vi "Main.vi"() -> ()   [LabVIEW 2015]
uses:
  TypeDefs/Queue Data.ctl
  SubVIs/App Data.vi
  SubVIs/App Strings.vi
  FGV/Timer Actions.ctl
  Global 1.vi
panel:
  out "Status 3":string
  out "Status 2":string
  in  "Period [s]":dbl
  in  "Device name":tag="myDAQ1"
  out "Time Elapsed":dbl format="%<%M:%S>t"
  out "Status":string
  in  "Time [ms]":dbl
  in  "Frequency":dbl
  in  "Stop Button":bool
  in  "Acquire Button":bool
  out "Waveform Graph":dbl[](graph)
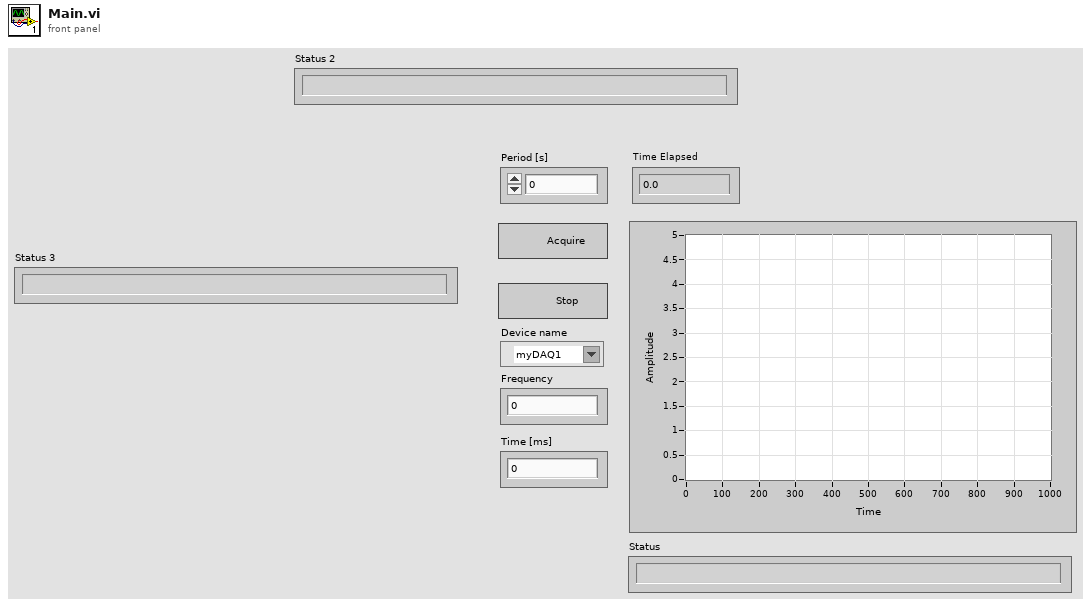
[diagram p1: front panel]
types:
  T1 = typedef "Timer Actions.ctl" = enum16{"Reset", "Get"}
  T2 = typedef "Queue Data.ctl" = cluster{"Action":string}
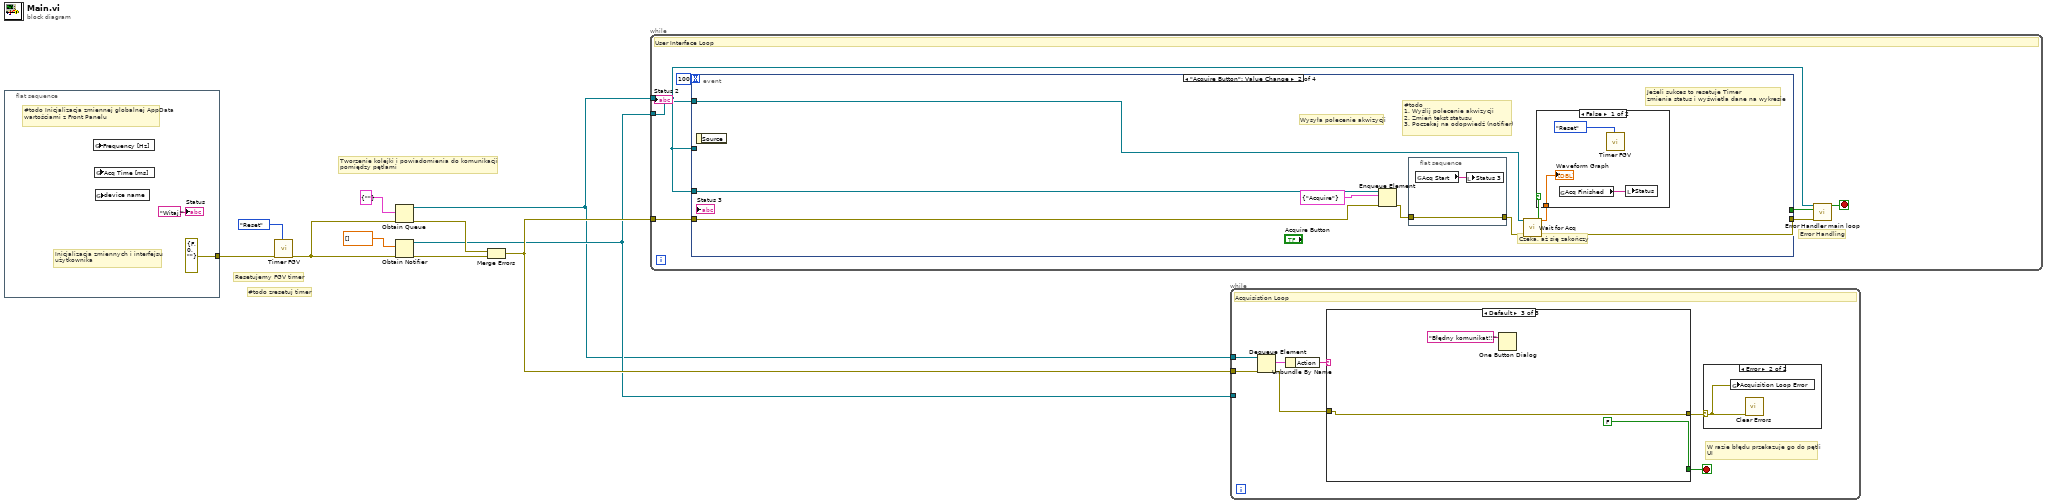
[diagram p0: block diagram]
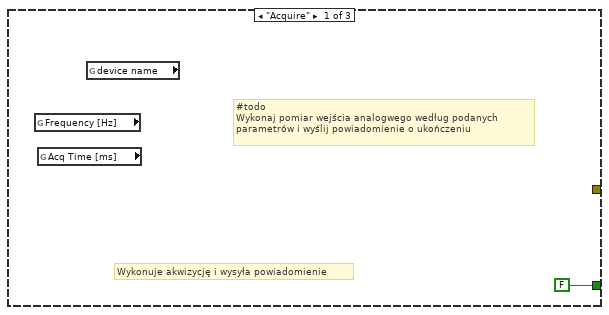
[diagram p3: hidden frame]
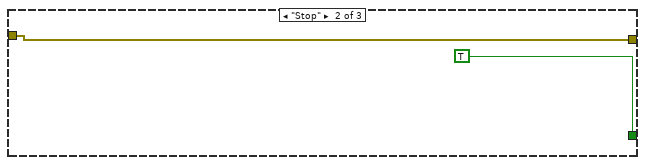
[diagram p4: hidden frame]
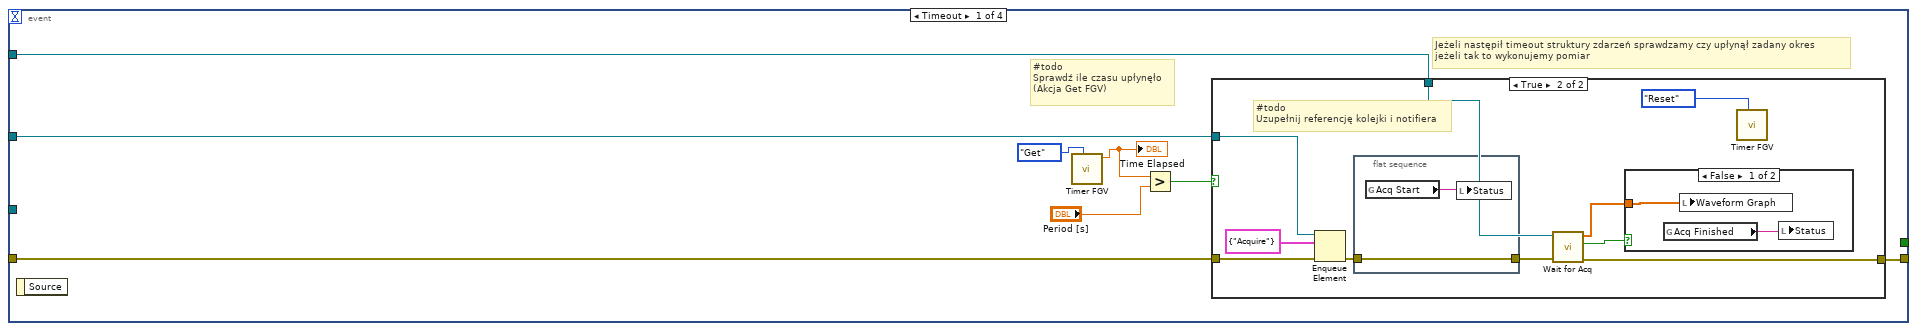
[diagram p5: hidden frame]
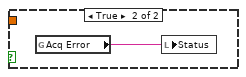
[diagram p7: hidden frame]
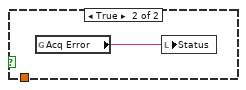
[diagram p8: hidden frame]
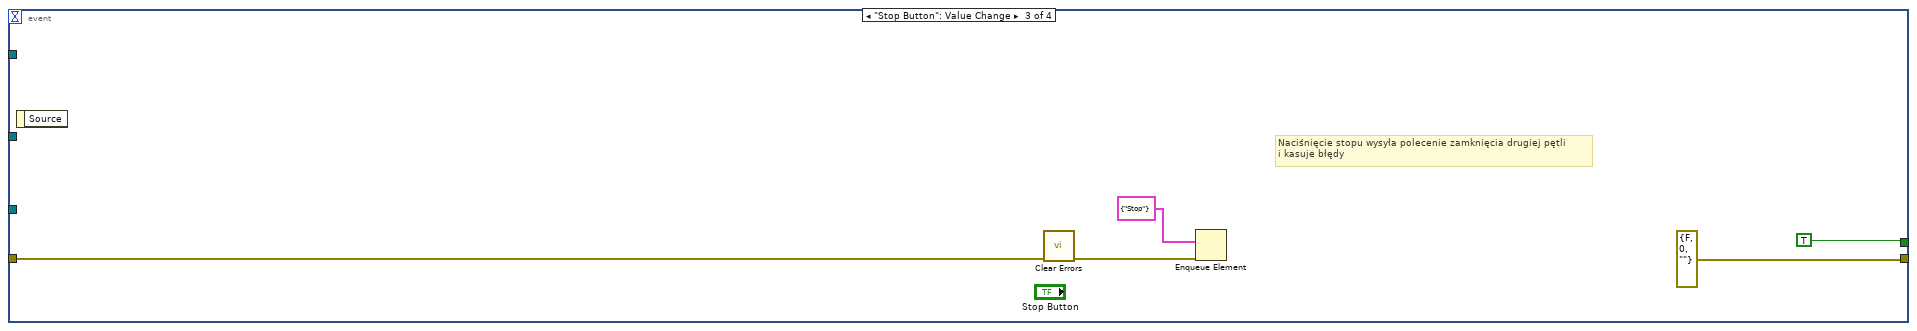
[diagram p9: hidden frame]
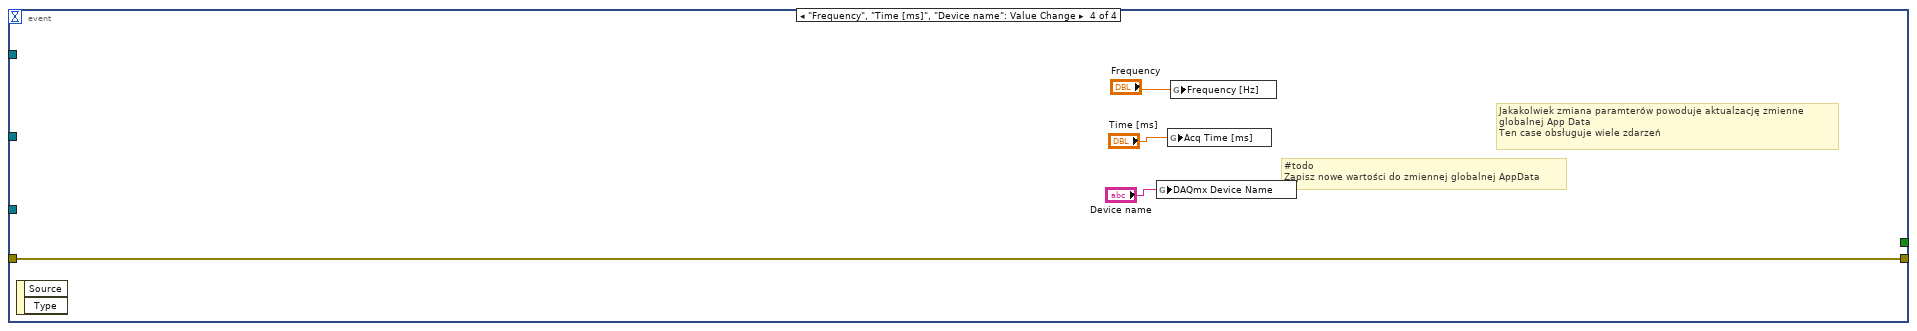
[diagram p10: hidden frame]
diagram:
  # "#todo zresetuj timer"
  # "Resetujemy FGV timer"
  # "Tworzenie kolejki i powiadomienia do komunikacji \npomiędzy pętlami"
  n1 = flat-sequence {
    tunnel: [errorcluster {"status"=FALSE, "code"=0, "source"=""} ("error constant")] -> w3
    frame #0 {
      # "#todo Inicjalizacja zmiennej globalnej AppData wartościami z Front Panelu"
      # "Inicjalizacja zmiennych i interfejsu \nużytkownika"
      n2 = global read "App Data.vi" "Frequency [Hz]"() -> ()  [unwired: 1 in]
      n3 = global read "App Data.vi" "Acq Time [ms]"() -> ()  [unwired: 1 in]
      n4 = global read "App Data.vi" "device name"() -> ()  [unwired: 1 in]
      "Status" <- "Witaj!" ("Status")
    }
  }
  n5 = call "Timer FGV.vi"("Action"=Timer_Actions."Reset", "error in (no error)"=w3) -> ("error out"=w2:errorcluster)  [unwired: 8 in, 1 out]
  n6 = Obtain Queue(element data type=T2 {"Action"=""}, error in (no error)=w2) -> (queue out=w4:refnum<queue>, error out=w9:errorcluster)  [unwired: 3 in, 1 out]
  n7 = Obtain Notifier(notification data type=dbl[] [], error in (no error)=w2) -> (notifier out=w5:refnum<notifier>, error out=w7:errorcluster)  [unwired: 2 in, 1 out]
  n8 = Merge Errors(w9, w7) -> (w6:errorcluster)
  n9 = while {
    tunnel: w6 -> [w18]
    tunnel: w4 -> [w14]
    tunnel: w5 -> [w13]
    stop <- w15 stop-if-true
    # "Error Handling"
    # "User Interface Loop"
    n10 = event shown="[1] \"Acquire Button\": Value Change" {
      selector: _ -> [_ _ _ _]
      dyn-events: _ -> [_ _ _ _]
      timeout: 100 -> [_ _ _ _]
      tunnel: w18 -> [w25 w50 w60 w67]
      tunnel: [w24 w45 errorcluster {"status"=FALSE, "code"=0, "source"=""} ("error constant") w67] -> w16
      tunnel: [_ _ TRUE _] -> w17
      tunnel: w14 -> [_ w52 _ _]
      tunnel: w14 -> [w23 _ _ _]
      tunnel: w13 -> [w20 w47 _ _]
      event Timeout {
        # "#todo\nSprawdź ile czasu upłynęło\n(Akcja Get FGV)"
        # "Jeżeli następił timeout struktury zdarzeń sprawdzamy czy upłynął zadany okres \njeżeli tak to wykonujemy pomiar"
        n11 = event-data() -> ()  [unwired: 1 in, 1 out]
        n12 = call "Timer FGV.vi"("Action"=Timer_Actions."Get") -> ("Elapsed Time"=w21:dbl)  [unwired: 9 in, 1 out]
        "Time Elapsed" <- w21
        n13 = Greater?(x=w21, y="Period [s]") -> (0:w26:bool)
        n14 = case shown="True" w26 {
          tunnel: w25 -> [w28 w38]
          tunnel: [w28 w31] -> w24
          tunnel: w23 -> [_ w30]
          tunnel: w20 -> [_ w29]
          frame False {
          }
          frame True {
            # "#todo\nUzupełnij referencję kolejki i notifiera"
            n15 = Enqueue Element(queue=w30, element=T2 {"Action"="Acquire"}, error in (no error)=w38) -> (error out=w36:errorcluster)  [unwired: 1 in, 2 out]
            n16 = flat-sequence {
              tunnel: w36 -> [w42]
              tunnel: [w42] -> w35
              frame #0 {
                n17 = global read "App Strings.vi" "Acq Start"() -> (w43:string)
                n18 = local write "Status"(w43) -> ()
              }
            }
            n19 = call "Wait for Acq.vi"("error in (no error)"=w35, "Notifier in"=w29) -> ("error out"=w31:errorcluster, "timed out?"=w32:bool, "Array"=w34:dbl[])  [unwired: 7 in]
            n20 = case shown="False" w32 {
              tunnel: w34 -> [w39 _]
              frame False {
                n21 = global read "App Strings.vi" "Acq Finished"() -> (w40:string)
                n22 = local write "Waveform Graph"(w39) -> ()
                n23 = local write "Status"(w40) -> ()
              }
              frame True {
                n24 = global read "App Strings.vi" "Acq Error"() -> (w41:string)
                n25 = local write "Status"(w41) -> ()
              }
            }
            n26 = call "Timer FGV.vi"("Action"=Timer_Actions."Reset") -> ()  [unwired: 9 in, 2 out]
          }
        }
      }
      event "Acquire Button": Value Change {
        # "#todo\n1. Wyślij polecenie akwizycji\n2. Zmień tekst statusu\n3. Poczekaj na odopwiedź (notifier)"
        # "Jeżeli sukces to resetuje Timer\nzmienia status i wyświetla dane na wykresie"
        # "Czeka, aż się zakończy"
        # "Wysyła polecenie akwizycji"
        n27 = event-data() -> ()  [unwired: 1 in, 1 out]
        n28 = Enqueue Element(queue=w52, element=T2 {"Action"="Acquire"}, error in (no error)=w50) -> (error out=w49:errorcluster)  [unwired: 1 in, 2 out]
        n29 = flat-sequence {
          tunnel: w49 -> [w53]
          tunnel: [w53] -> w46
          frame #0 {
            n30 = global read "App Strings.vi" "Acq Start"() -> (w54:string)
            n31 = local write "Status 3"(w54) -> ()
          }
        }
        n32 = call "Wait for Acq.vi"("error in (no error)"=w46, "Notifier in"=w47) -> ("error out"=w45:errorcluster, "timed out?"=w48:bool, "Array"=w44:dbl[])  [unwired: 7 in]
        n33 = case shown="False" w48 {
          tunnel: w44 -> [w55 _]
          frame False {
            n34 = global read "App Strings.vi" "Acq Finished"() -> (w57:string)
            n35 = call "Timer FGV.vi"("Action"=Timer_Actions."Reset") -> ()  [unwired: 9 in, 2 out]
            n36 = local write "Status"(w57) -> ()
            "Waveform Graph" <- w55
          }
          frame True {
            n37 = global read "App Strings.vi" "Acq Error"() -> (w58:string)
            n38 = local write "Status"(w58) -> ()
          }
        }
      }
      event "Stop Button": Value Change {
        # "Naciśnięcie stopu wysyła polecenie zamknięcia drugiej pętli\ni kasuje błędy"
        n39 = event-data() -> ()  [unwired: 1 in, 1 out]
        n40 = call <vilib>:"Clear Errors.vi"("error in (no error)"=w60) -> ("error out"=w59:errorcluster)  [unwired: 5 in, 1 out]
        n41 = Enqueue Element(element=T2 {"Action"="Stop"}, error in (no error)=w59) -> ()  [unwired: 2 in, 3 out]
      }
      event "Frequency", "Time [ms]", "Device name": Value Change {
        # "#todo \nZapisz nowe wartości do zmiennej globalnej AppData"
        # "Jakakolwiek zmiana paramterów powoduje aktualzację zmienne \nglobalnej App Data\nTen case obsługuje wiele zdarzeń"
        n42 = event-data() -> ()  [unwired: 1 in, 2 out]
        n43 = global write "Global 1.vi" "DAQmx Device Name"("Device name") -> ()
        n44 = global write "Global 1.vi" "Acq Time [ms]"("Time [ms]") -> ()
        n45 = global write "Global 1.vi" "Frequency [Hz]"("Frequency") -> ()
      }
    }
    n46 = call "Error Handler main loop.vi"("error in (no error)"=w16, "Exit?"=w17, "Queue in"=w14) -> ("Exit?"=w15:bool)  [unwired: 8 in]
  }
  n47 = while {
    tunnel: w6 -> [w72]
    tunnel: w4 -> [w71]
    tunnel: w5 -> [_]
    stop <- w69 stop-if-true
    # "W razie błędu przekazuje go do pętli\nUI"
    # "Acquisistion Loop"
    n48 = Dequeue Element(queue=w71, error in (no error)=w72) -> (element=w74:T2, error out=w70:errorcluster)  [unwired: 1 in, 2 out]
    n49 = Unbundle By Name(w74) -> ("Action"=w73:string)
    n50 = case shown="Default" w73 {
      tunnel: w70 -> [_ w77 w80]
      tunnel: [FALSE TRUE FALSE] -> w69
      tunnel: [_ w77 w80] -> w68
      frame "Acquire" {
        # "#todo\nWykonaj pomiar wejścia analogwego według podanych \nparametrów i wyślij powiadomienie o ukończeniu"
        # "Wykonuje akwizycję i wysyła powiadomienie"
        n51 = global read "App Data.vi" "Frequency [Hz]"() -> ()  [unwired: 1 out]
        n52 = global read "App Data.vi" "Acq Time [ms]"() -> ()  [unwired: 1 out]
        n53 = global read "App Data.vi" "device name"() -> ()  [unwired: 1 out]
      }
      frame "Stop" {
      }
      frame Default {
        n54 = One Button Dialog(message="Błędny komunikat!!!") -> ()  [unwired: 1 in, 1 out]
      }
    }
    n55 = case shown="Error" w68 {
      selector: w68 -> [_ w75]
      frame No Error {
      }
      frame Error {
        n56 = global write "App Data.vi" "Acquisition Loop Error"(w75) -> ()
        n57 = call <vilib>:"Clear Errors.vi"("error in (no error)"=w75) -> ()  [unwired: 5 in, 2 out]
      }
    }
  }
